vi "Step(Tape).vi"(7 "downramp array":dbl[](array[numeric]), 8 "error in (no error)":errorcluster, 10 "Settings":T1={"max velocity"={"Value"=0.0, "Min"=0.0, "Max"=0.0, "StepSize"=0.0, "Tolerance"=0.0, "ValueActual"=0.0}, "continious velocity"={"Value"=0.0, "Min"=0.0, "Max"=0.0, "StepSize"=0.0, "Tolerance"=0.0, "ValueActual"=0.0}, "shake"=enum."off", "direction"=enum."left", "RedRatio"={"Value"=0.0, "Min"=0.0, "Max"=0.0, "StepSize"=0.0, "Tolerance"=0.0, "ValueActual"=0.0}, "StepSize"={"Value"=0.0, "Min"=0.0, "Max"=0.0, "StepSize"=0.0, "Tolerance"=0.0, "ValueActual"=0.0}, "position"={"Value"=0.0, "Min"=0.0, "Max"=0.0, "StepSize"=0.0, "Tolerance"=0.0, "ValueActual"=0.0}, "velocity"={"Value"=0.0, "Min"=0.0, "Max"=0.0, "StepSize"=0.0, "Tolerance"=0.0, "ValueActual"=0.0}, "Step"=enum."off", "Mode"=enum."on demand", "timeout"={"Value"=0.0, "Min"=0.0, "Max"=0.0, "StepSize"=0.0, "Tolerance"=0.0, "ValueActual"=0.0}, "DelayStage"={"Value"=0.0, "Min"=0.0, "Max"=0.0, "StepSize"=0.0, "Tolerance"=0.0, "ValueActual"=0.0}, "TapeMotor"=enum."off", "encoder Axis"=2, "oldpos"=0.0, "ResetEncoder"=enum."off", "ignore tape monitor"=enum."off"}, 11 "VISA resource name":refnum<visa-resource-name>) -> (0 "error out":errorcluster, 1 "trajectories":dbl[][](graph)=[[1.0, 0.7046880791959296, 0.4965852858533471, 0.3499377259476329, 0.2465969370957652, 0.1737739140097176, 0.12245639698366893, 0.08629355394147512, 0.06081002915927391, 0.0628100291592739, 0.0648100291592739, 0.0668100291592739, 0.06881002915927391, 0.08881002915927391, 0.12881002915927392, 0.18881002915927392, 0.26881002915927393, 0.36881002915927397, 0.48881002915927396, 0.628810029159274, 0.788810029159274, 0.968810029159274, 1.0], [0.0, 0.0, 0.0, 0.0, 0.0, 0.0, 0.004000000000814907, 0.002999999998792191, 0.040000000000873115, 0.20499999999992724, 0.363999999999578, 0.5879999999997381, 0.7160000000003492, 0.7360000000007858, 0.7879999999986467, 0.6760000000012951, 0.3989999999994325, 0.01300000000082946, 0.004000000000814907, 0.003999999998995918, 0.0, 0.0, 0.0], [0.0, 0.0, 0.0, 0.0, 0.0, 0.0, 0.004000000000814907, -0.0010000000020227162, 0.037000000002080924, 0.16499999999905413, 0.15899999999965075, 0.22400000000016007, 0.12800000000061118, 0.020000000000436557, 0.05199999999786087, -0.11199999999735155, -0.27700000000186265, -0.385999999998603, -0.009000000000014552, -1.8189894035458565e-12, -0.003999999998995918, 0.0, 0.0]], 2 "Settings":T1={"max velocity"={"Value"=0.0, "Min"=0.0, "Max"=0.0, "StepSize"=0.0, "Tolerance"=0.0, "ValueActual"=0.0}, "continious velocity"={"Value"=0.0, "Min"=0.0, "Max"=0.0, "StepSize"=0.0, "Tolerance"=0.0, "ValueActual"=0.0}, "shake"=enum."off", "direction"=enum."left", "RedRatio"={"Value"=0.0, "Min"=0.0, "Max"=0.0, "StepSize"=0.0, "Tolerance"=0.0, "ValueActual"=0.0}, "StepSize"={"Value"=0.0, "Min"=0.0, "Max"=0.0, "StepSize"=0.0, "Tolerance"=0.0, "ValueActual"=0.0}, "position"={"Value"=0.0, "Min"=0.0, "Max"=0.0, "StepSize"=0.0, "Tolerance"=0.0, "ValueActual"=0.0}, "velocity"={"Value"=0.0, "Min"=0.0, "Max"=0.0, "StepSize"=0.0, "Tolerance"=0.0, "ValueActual"=0.0}, "Step"=enum."off", "Mode"=enum."on demand", "timeout"={"Value"=0.0, "Min"=0.0, "Max"=0.0, "StepSize"=0.0, "Tolerance"=0.0, "ValueActual"=0.0}, "DelayStage"={"Value"=0.0, "Min"=0.0, "Max"=0.0, "StepSize"=0.0, "Tolerance"=0.0, "ValueActual"=0.0}, "TapeMotor"=enum."off", "encoder Axis"=2, "oldpos"=0.0, "ResetEncoder"=enum."off", "ignore tape monitor"=enum."off"}, 3 "VISA resource name out":refnum<visa-resource-name>, 4 "ok":bool, 5 "position":dbl)   [LabVIEW 2013]
uses:
  settings_TypDef.ctl
  shared/numericVariable_TypeDef.ctl
  shared/OnOffTypeDef.ctl
  Direction_TypDef.ctl
  Mode_TypDEf.ctl
  shared/CompressAndUpdate(Poly)/CompressAndUpdate(Numeric).vi
  Newport ESP301/Newport ESP301.lvlib
  BaseDriver/BaseDriver.lvclass
  TapeDrive.lvclass
panel:
  out "Position (units)":dbl(graph)=-13329.169
  out "velocity":dbl(graph)
  out "ratio":dbl(graph)=1.0
  out "acceleration":dbl(graph)
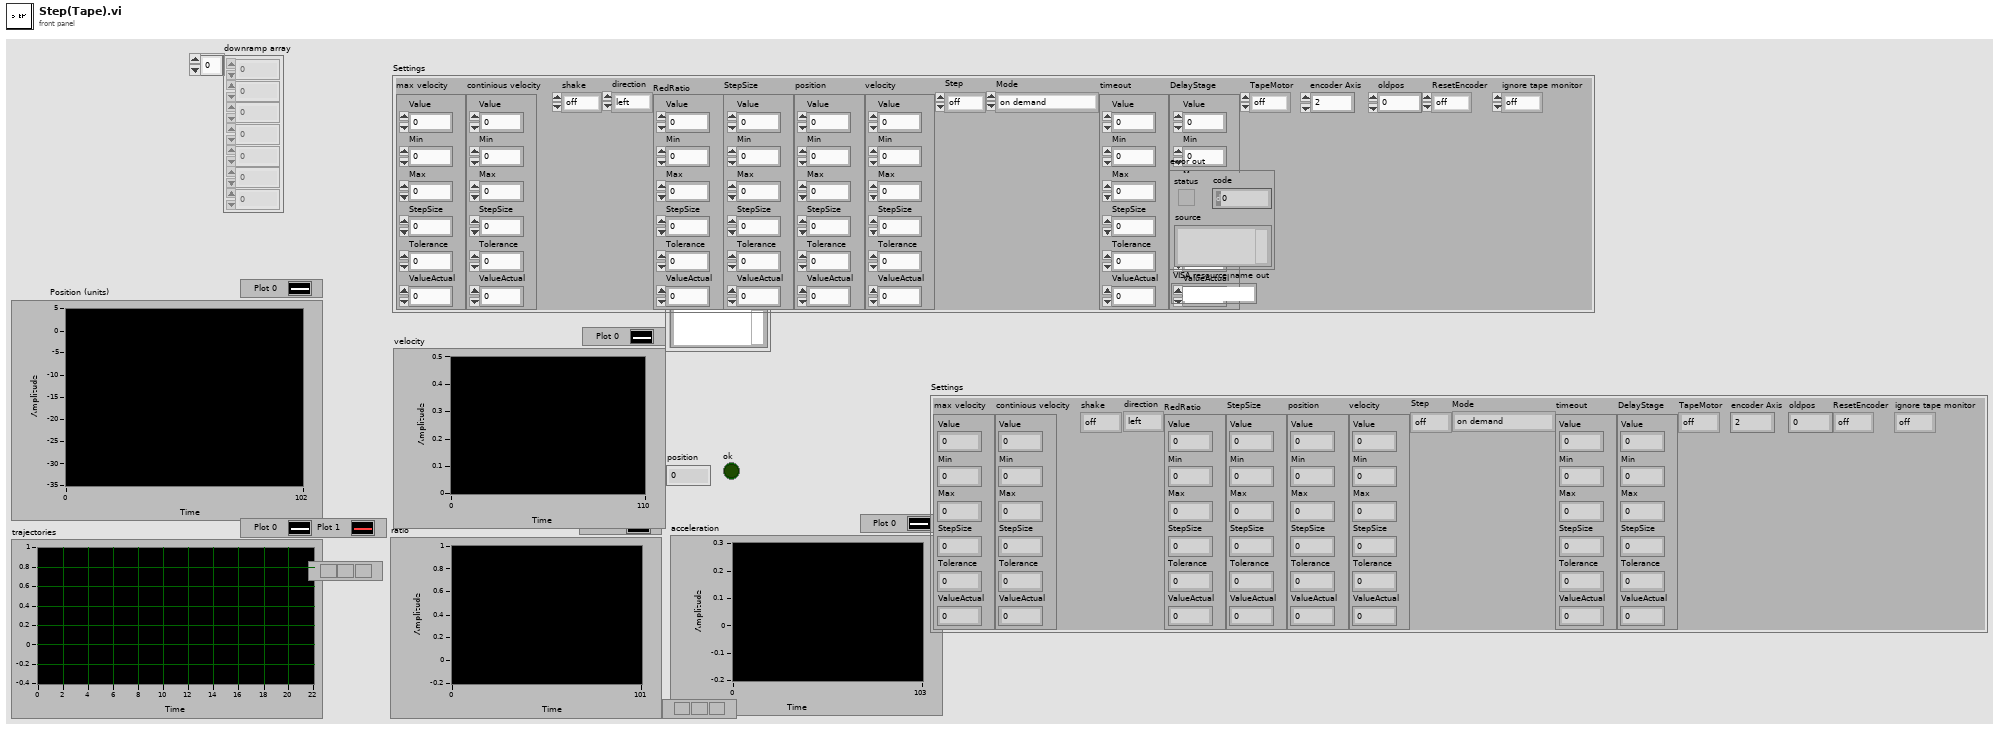
[diagram p1: front panel]
types:
  T1 = typedef "TapeDrive.lvclass/settings_TypDef.ctl" = cluster{"max velocity":T2, "continious velocity":T2, "shake":T3, "direction":T4, "RedRatio":T2, "StepSize":T2, "position":T2, "velocity":T2, "Step":T3, "Mode":T5, "timeout":T2, "DelayStage":T2, "TapeMotor":T3, "encoder Axis":i32, "oldpos":dbl, "ResetEncoder":T3, "ignore tape monitor":T3}
  T2 = typedef "BaseDriver.lvclass/numericVariable_TypeDef.ctl" = cluster{"Value":dbl, "Min":dbl, "Max":dbl, "StepSize":dbl, "Tolerance":dbl, "ValueActual":dbl}
  T3 = typedef "OnOffTypeDef.ctl" = enum16{"off", "on"}
  T4 = typedef "Direction_TypDef.ctl" = enum16{"left", "right"}
  T5 = typedef "Mode_TypDEf.ctl" = enum16{"on demand", "continuous", "scan"}
  T6 = cluster{"increase":dbl, "min velocity":dbl, "max velocity":dbl, "Stop increase":dbl}
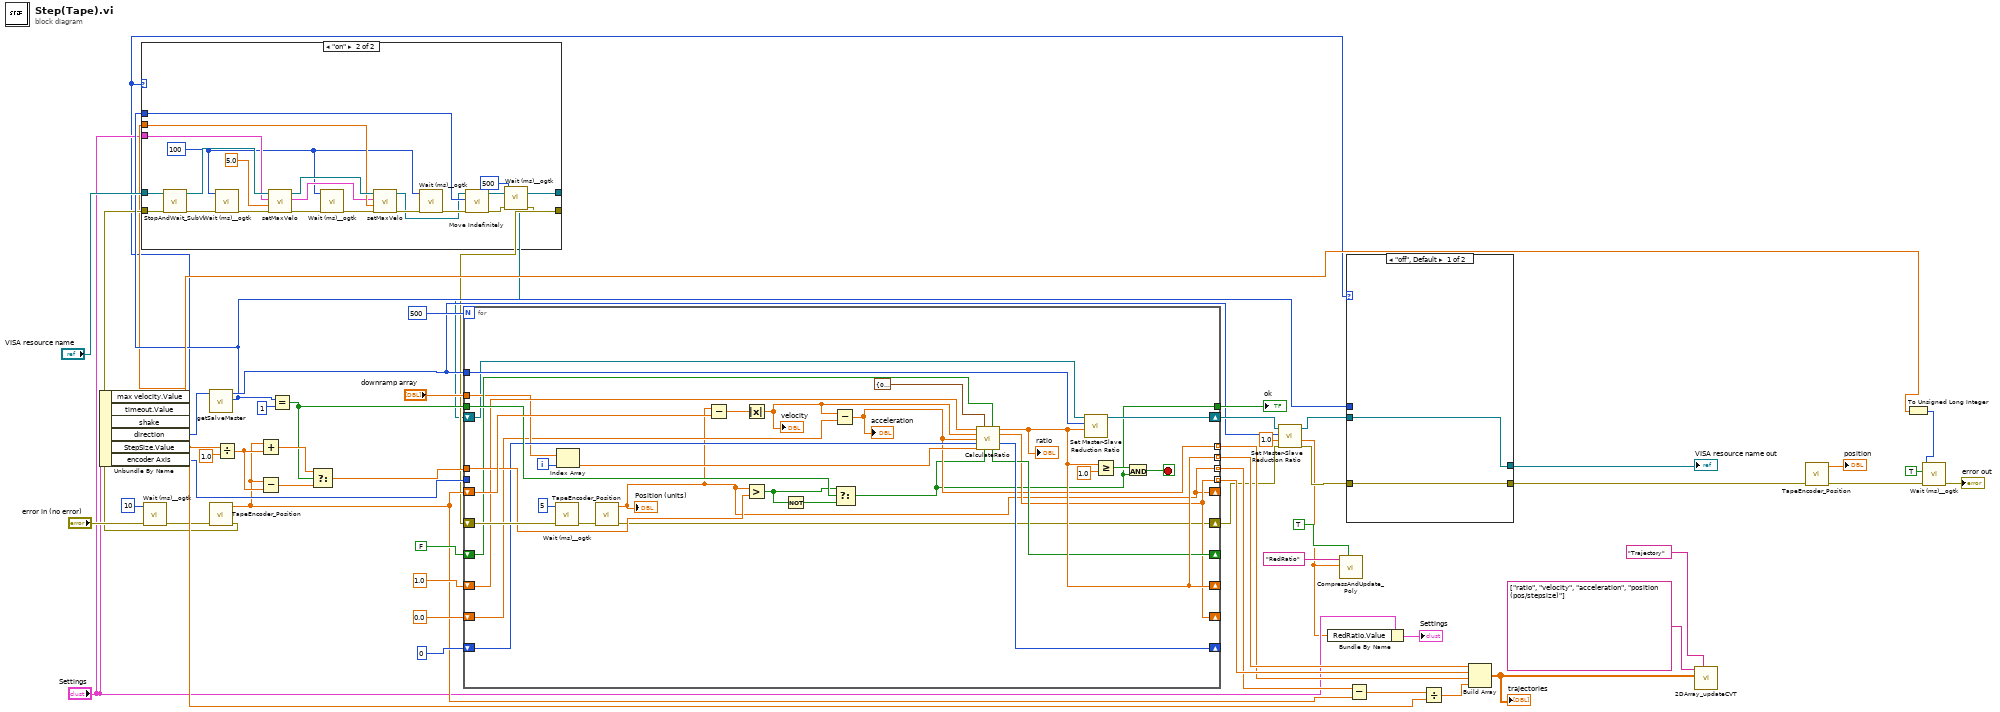
[diagram p0: block diagram]
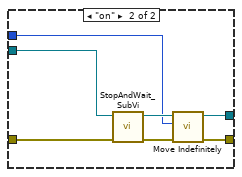
[diagram p3: hidden frame]
diagram:
  w3 = 1.0 ("Reduction Ratio (0)")
  n1 = Unbundle By Name("Settings") -> ("max velocity.Value"=w5:dbl, "timeout.Value"=w16:dbl, "shake"=w1:T3, "direction"=w38:T4, "StepSize.Value"=w31:dbl, "encoder Axis"=w23:i32)
  n2 = call <userlib>:"Wait (ms)__ogtk.vi"("error in (no error)"="error in (no error)", "milliseconds to wait"=u32 10) -> ("error out"=w22:errorcluster)  [unwired: 8 in, 1 out]
  n3 = call "TapeEncoder_Position.vi"("error in (no error)"=w22) -> ("error IO"=w7:errorcluster, "position"=w21:dbl)  [unwired: 9 in]
  n4 = call "getSalveMaster.vi"("direction"=w38) -> ("Master"=w8:i32, "Slave"=w12:i32)  [unwired: 9 in]
  n5 = case shown="\"on\"" w1 {
    tunnel: "VISA resource name" -> [w57 w78]
    tunnel: [w57 w77] -> w2
    tunnel: w8 -> [_ w76]
    tunnel: w7 -> [w56 w75]
    tunnel: [w56 w60] -> w6
    tunnel: w5 -> [_ w64]
    tunnel: "Settings" -> [_ w63]
    frame "off", Default {
    }
    frame "on" {
      w59 = u32 100 ("milliseconds to wait")
      n6 = call "StopAndWait_SubVi.vi"("error in (no error)"=w75, "VISA Refnum in"=w78) -> ("error out"=w74:errorcluster, "VISA Refnum out"=w73:refnum<visa-resource-name>)  [unwired: 8 in]
      n7 = call <userlib>:"Wait (ms)__ogtk.vi"("error in (no error)"=w74, "milliseconds to wait"=w59) -> ("error out"=w72:errorcluster)  [unwired: 8 in, 1 out]
      n8 = call "setMaxVelo.vi"("error in (no error)"=w72, "NewVal"=5.0, "Settings"=w63, "VISA Refnum in"=w73) -> ("error out"=w70:errorcluster, "Settings"=w62:T1, "VISA Refnum out"=w66:refnum<visa-resource-name>)  [unwired: 4 in, 1 out]
      n9 = call <userlib>:"Wait (ms)__ogtk.vi"("error in (no error)"=w70, "milliseconds to wait"=w59) -> ("error out"=w69:errorcluster)  [unwired: 8 in, 1 out]
      n10 = call "setMaxVelo.vi"("error in (no error)"=w69, "NewVal"=w64, "Settings"=w62, "VISA Refnum in"=w66) -> ("error out"=w68:errorcluster, "VISA Refnum out"=w65:refnum<visa-resource-name>)  [unwired: 4 in, 2 out]
      n11 = call <userlib>:"Wait (ms)__ogtk.vi"("error in (no error)"=w68, "milliseconds to wait"=w59) -> ("error out"=w67:errorcluster)  [unwired: 8 in, 1 out]
      n12 = call "Move Indefinitely.vi"("error in (no error)"=w67, "Axis (1)"=w76, "VISA resource name"=w65) -> ("error out"=w61:errorcluster, "VISA resource name out"=w77:refnum<visa-resource-name>)  [unwired: 3 in]
      n13 = call <userlib>:"Wait (ms)__ogtk.vi"("error in (no error)"=w61, "milliseconds to wait"=u32 500) -> ("error out"=w60:errorcluster)  [unwired: 8 in, 1 out]
    }
  }
  n14 = Divide(x=w31, y=1.0) -> (x/y=w43:dbl)
  n15 = Add(x=w21, y=w43) -> (x+y=w52:dbl)
  n16 = Subtract(x=w21, y=w43) -> (x-y=w51:dbl)
  n17 = Equal?(x=w8, y=1) -> (x = y?=w49:bool)
  n18 = Select(t=w52, s=w49, f=w51) -> (s? t:f=w50:dbl)
  n19 = for {
    N: 500 -> [_]
    shift-right: [w81] -> w11
    shift-left: w6 -> [w108]
    tunnel: w12 -> [w109]
    shift-right: [w80] -> _
    shift-left: w21 -> [w106]
    shift-right: [w97] -> _
    shift-left: 1.0 -> [w96]
    tunnel: w50 -> [w104]
    tunnel: w49 -> [w102]
    shift-right: [w98] -> _
    shift-left: 0 -> [w99]
    tunnel: [w97] -> w47 mode=indexing
    tunnel: [w86] -> w46 mode=indexing
    tunnel: "downramp array" -> [w91]
    shift-right: [w92] -> _
    shift-left: FALSE -> [w93]
    shift-right: [w86] -> _
    shift-left: 0.0 -> [w87]
    tunnel: [w85] -> w39 mode=indexing
    tunnel: [w80] -> w33 mode=indexing
    tunnel: [w83] -> w24
    tunnel: w23 -> [_]
    shift-right: [w110] -> w14
    shift-left: w2 -> [w79]
    i -> [w90]
    stop <- w94 stop-if-true
    n20 = call <userlib>:"Wait (ms)__ogtk.vi"("error in (no error)"=w108, "milliseconds to wait"=u32 5) -> ("error out"=w82:errorcluster)  [unwired: 8 in, 1 out]
    n21 = Index Array(array=w91, index=w90) -> (element=w89:dbl)
    n22 = call "TapeEncoder_Position.vi"("error in (no error)"=w82) -> ("error IO"=w81:errorcluster, "position"=w80:dbl)  [unwired: 9 in]
    "Position (units)" <- w80
    n23 = Subtract(x=w80, y=w106) -> (x-y=w105:dbl)
    n24 = Absolute Value(x=w105) -> (abs(x)=w88:dbl)
    "velocity" <- w88
    n25 = Greater?(x=w80, y=w104) -> (0:w100:bool)
    n26 = Not(x=w100) -> (.not. x?=w101:bool)
    n27 = Subtract(x=w88, y=w87) -> (x-y=w85:dbl)
    "acceleration" <- w85
    n28 = Select(t=w100, s=w102, f=w101) -> (s? t:f=w83:bool)
    n29 = call "CalculateRatio.vi"("ratio"=w96, "Cluster"=T6 {"increase"=0.004, "min velocity"=0.1, "max velocity"=3.0, "Stop increase"=0.02}, "decrease again"=w93, "velocity"=w88, "acceleration"=w85, "rep"=w99, "downramp"=w89, "stop"=w83) -> ("ratio out"=w97:dbl, "velocity out"=w86:dbl, "rep out"=w98:i32, "decrease again out"=w92:bool)  [unwired: 4 in]
    "ratio" <- w97
    n30 = call "Set Master-Slave Reduction Ratio.vi"("Reduction Ratio (0)"=w97, "Axis (1)"=w109, "VISA resource name"=w79) -> ("VISA resource name out"=w110:refnum<visa-resource-name>)  [unwired: 3 in, 1 out]
    n31 = Greater Or Equal?(x=w97, y=1.0) -> (x >= y?=w95:bool)
    n32 = And(x=w95, y=w83) -> (x .and. y?=w94:bool)
  }
  "ok" <- w24
  n33 = call "Set Master-Slave Reduction Ratio.vi"("error in (no error)"=w11, "Reduction Ratio (0)"=w3, "Axis (1)"=w12, "VISA resource name"=w14) -> ("error out"=w10:errorcluster, "VISA resource name out"=w13:refnum<visa-resource-name>)  [unwired: 2 in]
  n34 = Bundle By Name(cluster="Settings", "RedRatio.Value"=w3) -> (→"Settings":T1)
  n35 = call-poly "CompressAndUpdate_Poly.vi"("force CVT update (false)"=TRUE, "Numeric"=w3, "command or variable name"="RedRatio") -> ()  [unwired: 8 in, 1 out]
  n36 = case shown="\"off\", Default" w1 {
    tunnel: w13 -> [w112 w119]
    tunnel: [w112 w117] -> w45
    tunnel: w8 -> [_ w116]
    tunnel: w10 -> [w111 w115]
    tunnel: [w111 w113] -> w20
    frame "off", Default {
    }
    frame "on" {
      n37 = call "StopAndWait_SubVi.vi"("error in (no error)"=w115, "VISA Refnum in"=w119) -> ("error out"=w114:errorcluster, "VISA Refnum out"=w118:refnum<visa-resource-name>)  [unwired: 8 in]
      n38 = call "Move Indefinitely.vi"("error in (no error)"=w114, "Axis (1)"=w116, "VISA resource name"=w118) -> ("error out"=w113:errorcluster, "VISA resource name out"=w117:refnum<visa-resource-name>)  [unwired: 3 in]
    }
  }
  "VISA resource name out" <- w45
  n39 = Subtract(x=w33, y=w21) -> (x-y=w32:dbl[])
  n40 = Divide(x=w32, y=w31) -> (x/y=w30:dbl[])
  n41 = Build Array(w47, w46, w39, w30) -> (w28:dbl[][])
  "trajectories" <- w28
  n42 = call "2DArray_updateCVT.vi"("CVt_clusterName"="Trajectory", "trajectories"=w28, "Names"=string[] ["ratio", "velocity", "acceleration", "position (pos/stepsize)"]) -> ()  [unwired: 8 in, 1 out]
  n43 = call "TapeEncoder_Position.vi"("error in (no error)"=w20) -> ("error IO"=w19:errorcluster, "position"=→"position":dbl)  [unwired: 9 in]
  n44 = To Unsigned Long Integer(number=w16) -> (unsigned 32bit integer=w15:u32)
  n45 = call <userlib>:"Wait (ms)__ogtk.vi"("error in (no error)"=w19, "Wait on Error (FALSE)"=TRUE, "milliseconds to wait"=w15) -> ("error out"=→"error out":errorcluster)  [unwired: 7 in, 1 out]
